vi "CountShots.vi"(1 "Shooter Goal (rpm)":dbl, 2 "Shooter Velocity (rpm)":dbl) -> (0 "Number of Balls Shot":i32)   [LabVIEW 2019]
panel:
  in  "Count Delta (rpm)":dbl=200.0
  in  "Arm Delta (rpm)":dbl=100.0
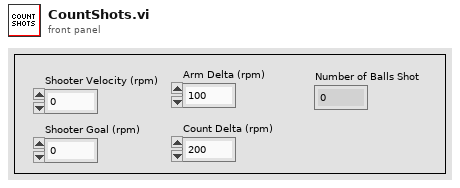
[diagram p1: front panel]
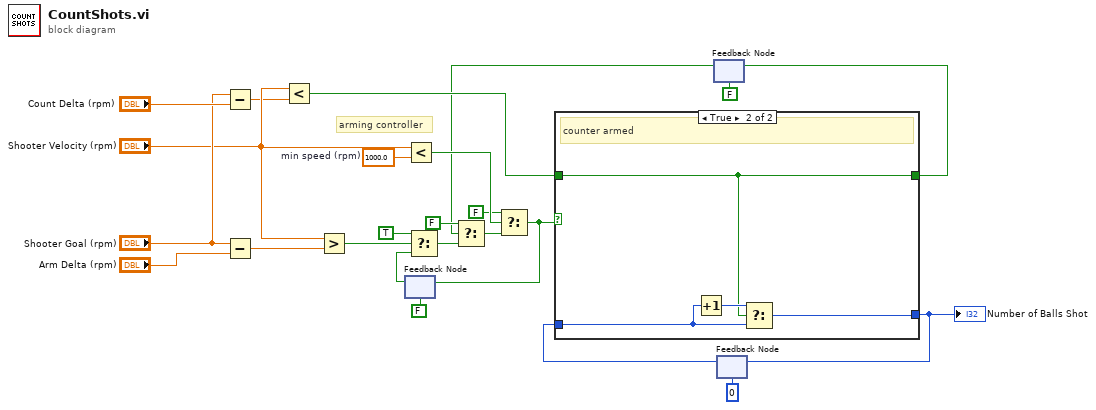
[diagram p0: block diagram]
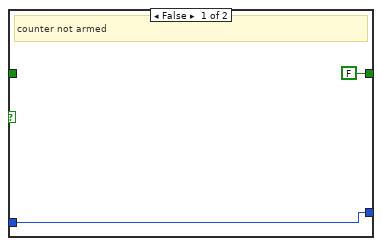
[diagram p2: hidden frame]
diagram:
  w16 = 1000.0  # min speed (rpm)
  # "arming controller"
  n1 = Subtract(x="Shooter Goal (rpm)", y="Count Delta (rpm)") -> (x-y=w5:dbl)
  n2 = Subtract(x="Shooter Goal (rpm)", y="Arm Delta (rpm)") -> (x-y=w23:dbl)
  n3 = Less?(x="Shooter Velocity (rpm)", y=w5) -> (x < y?=w4:bool)
  n4 = Greater?(x="Shooter Velocity (rpm)", y=w23) -> (0:w22:bool)
  n5 = feedback #1(FALSE) -> (w20:bool)
  n6 = Less?(x="Shooter Velocity (rpm)", y=w16) -> (x < y?=w15:bool)
  n7 = Select(t=TRUE, s=w22, f=w20) -> (s? t:f=w18:bool)
  n8 = feedback #2(FALSE) -> (w1:bool)
  n9 = Select(t=FALSE, s=w1, f=w18) -> (s? t:f=w17:bool)
  n10 = Select(t=FALSE, s=w15, f=w17) -> (s? t:f=w13:bool)
  n11 = feedback-in #1(w13) -> ()
  n12 = feedback #3(0) -> (w11:i32)
  n13 = case shown="True" w13 {
    tunnel: w11 -> [w26 w29]
    tunnel: [w26 w30] -> w10
    tunnel: w4 -> [_ w27]
    tunnel: [FALSE w27] -> w3
    frame False {
      # "counter not armed"
    }
    frame True {
      # "counter armed"
      n14 = Increment(x=w29) -> (x+1=w28:i32)
      n15 = Select(t=w28, s=w27, f=w29) -> (s? t:f=w30:i32)
    }
  }
  "Number of Balls Shot" <- w10
  n16 = feedback-in #2(w3) -> ()
  n17 = feedback-in #3(w10) -> ()
